vi "Serial Close IMU.vi"(8 "error out":errorcluster, 11 "FPGA IMU IN 2":refnum<k20>) -> (0 "error out":errorcluster)   [LabVIEW 2016]
uses:
  <vilib>/rvi/interface/nirviReadWriteControl/nirviReadWriteControl.xnode
  <vilib>/rvi/interface/nirviCloseFPGA/nirviCloseFPGA.xnode
  FPGA Bitfiles/FPGAIMU_FPGATarget_FPGAIMURead_c-b2E2IVPMQ.lvbitx
  <vilib>/rvi/errors/niLvFpgaMergeErrorWithErrorCode.vi
  <vilib>/rvi/errors/niLvFpgaAdjustHostInterfaceError.vi
  <vilib>/FPGAPlugInAG/roboRIO/niLvFpga_Close_roboRIO.vi
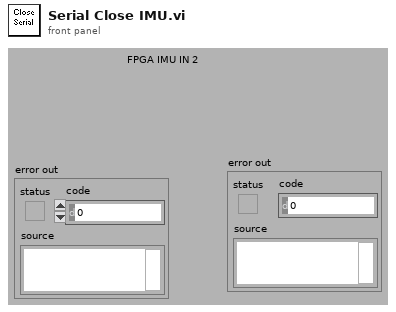
[diagram p1: front panel]
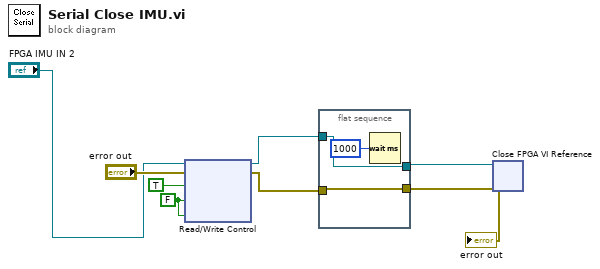
[diagram p0: block diagram]
diagram:
  w1 = FALSE ("Stop imu")
  n1 = xnode "Read/Write Control"("FPGA VI Reference In"="FPGA IMU IN 2", "error in"="error out", "stop"=TRUE, "Stop imu"=w1, "Start imu"=w1) -> ("FPGA VI Reference Out"=w5:refnum<k20>, "error out"=w4:errorcluster)
  n2 = flat-sequence {
    tunnel: w5 -> [w12]
    tunnel: [w12] -> w2
    tunnel: w4 -> [w11]
    tunnel: [w11] -> w3
    frame #0 {
      n3 = Wait (ms)(milliseconds to wait=u32 1000) -> ()  [unwired: 1 out]
    }
  }
  n4 = xnode "Close FPGA VI Reference"("FPGA VI Reference In"=w2, "error in"=w3) -> ("error out"=→"error out":errorcluster)
